vi "ep_Rectified and DC Values.vi"(8 "error in (no error)":errorcluster, 11 "data":waveform(dbl)[](array[waveform])) -> (0 "error out":errorcluster, 1 "calibrated ARVs":dbl[](array[numeric]), 2 "ARVs":dbl[](array[numeric]), 3 "DC values":dbl[](array[numeric]))   [LabVIEW 2024]
doc: "Calculates the average rectified values and DC values of input signals."
uses:
  <vilib>/Analysis/baseanly.llb/Mean (DBL).vi
  <vilib>/Analysis/NI_AALBase.lvlib
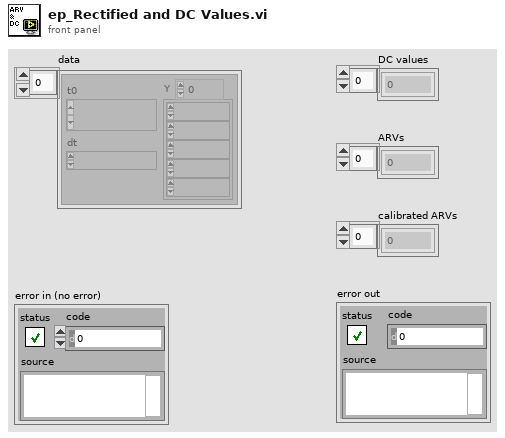
[diagram p1: front panel]
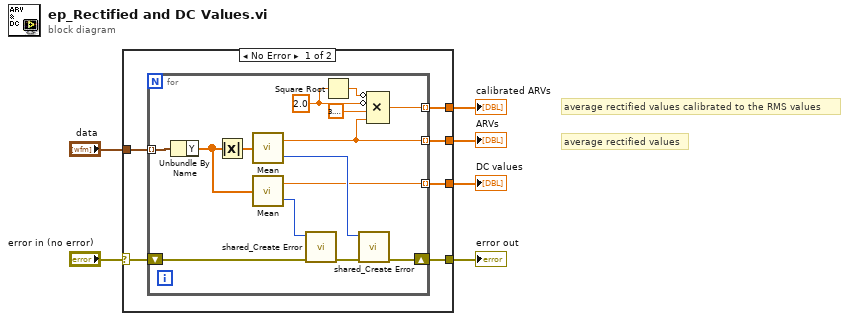
[diagram p0: block diagram]
diagram:
  # "average rectified values calibrated to the RMS values"
  # "average rectified values"
  n1 = case shown="No Error" "error in (no error)" {
    selector: "error in (no error)" -> [w11 w27]
    tunnel: "data" -> [w12 _]
    tunnel: [w10 _] -> w3
    tunnel: [w9 w27] -> w4
    tunnel: [w8 _] -> w2
    tunnel: [w7 _] -> w1
    frame No Error {
      n2 = for {
        tunnel: w12 -> [w26] mode=indexing
        shift-right: [w23] -> w9
        shift-left: w11 -> [w25]
        tunnel: [w18] -> w10 mode=indexing
        tunnel: [w17] -> w8 mode=indexing
        tunnel: [w13] -> w7 mode=indexing
        w16 = 2.0
        n3 = Unbundle By Name(w26) -> ("Y"=w20:dbl[])
        n4 = Absolute Value(x=w20) -> (abs(x)=w19:dbl[])
        n5 = call-poly <vilib>:"Mean.vi"("X"=w19) -> ("mean"=w17:dbl, "error"=w21:i32)
        n6 = call-poly <vilib>:"Mean.vi"("X"=w20) -> ("mean"=w18:dbl, "error"=w22:i32)
        n7 = call <vilib>:"shared_Create Error.vi"("error in (no error)"=w25, "error code (0)"=w22) -> ("error out"=w24:errorcluster)  [unwired: 9 in]
        n8 = Square Root(x=w16) -> (sqrt(x)=w15:dbl)
        n9 = call <vilib>:"shared_Create Error.vi"("error in (no error)"=w24, "error code (0)"=w21) -> ("error out"=w23:errorcluster)  [unwired: 9 in]
        n10 = Compound Arithmetic op=MULTIPLY(invert w15, invert w16, 3.141592653589793, w17) -> (w13:dbl)
      }
    }
    frame Error {
    }
  }
  "error out" <- w4
  "DC values" <- w3
  "ARVs" <- w2
  "calibrated ARVs" <- w1
